vi "Constructor.vi"(8 "error in (no error)":errorcluster, 10 "FilePath":path, 11 "Name":string) -> (0 "error out":errorcluster, 3 "DocumentType out":refnum<class "Document.lvclass">)   [LabVIEW 2021, in "ProligentXMLGenerator.lvlib" / "Document.lvclass"]
uses:
  Document.lvclass
  Data.ctl
  CustomData/CustomData.lvclass
  Base/Guid/Guid.lvclass
  Base/NonEmptyString_255/NonEmptyString_255.lvclass
  Base/NonNullableString_600/NonNullableString_600.lvclass
  Document.lvclass/Document.ctl
  SetFilePath.vi
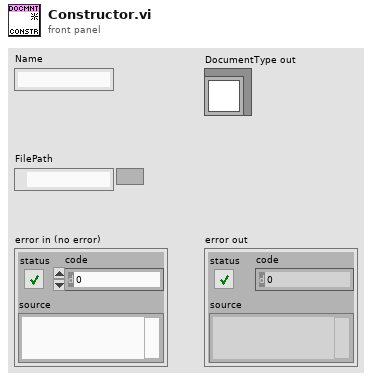
[diagram p1: front panel]
types:
  T1 = typedef "ProligentXMLGenerator.lvlib/Document.lvclass/Data.ctl" = cluster{"Name":string, "CustomData":refnum<class "CustomData.lvclass">, "Identifier":refnum<class "Guid.lvclass">, "NameType":refnum<class "NonEmptyString_255.lvclass">, "FileName":refnum<class "NonEmptyString_255.lvclass">, "Description":refnum<class "NonNullableString_600.lvclass">, "FilePath":path, "DestinationFolder":path}
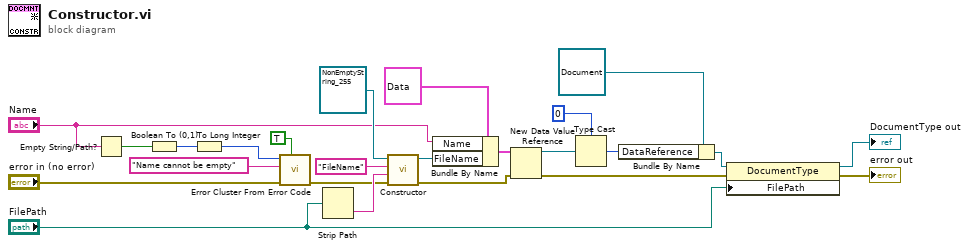
[diagram p0: block diagram]
diagram:
  n1 = Empty String/Path?(string/path="Name") -> (empty?=w24:bool)
  n2 = Boolean To (0,1)(Boolean=w24) -> (0, 1=w23:i16)
  n3 = To Long Integer(number=w23) -> (32bit integer=w17:i32)
  n4 = call <vilib>:"Error Cluster From Error Code.vi"("show call chain? (False)"=TRUE, "error in (no error)"="error in (no error)", "error message (\"\")"="Name cannot be empty" ("error message (\"\")"), "error code (0)"=w17) -> ("error out"=w13:errorcluster)  [unwired: 5 in]
  n5 = Strip Path(path="FilePath") -> (name=w18:string)  [unwired: 1 out]
  n6 = call-dynamic "Constructor.vi"("error in"=w13, "Value"=w18, "Name"="FileName", "String in"=refnum<class "NonEmptyString_255.lvclass"> refnum ("ProligentResultProcessor:NonEmptyString_255")) -> ("error out"=w3:errorcluster, "String out"=w21:refnum<class "NonEmptyString_255.lvclass">)  [unwired: 6 in]
  n7 = Bundle By Name(cluster=T1 {"Name"="", "CustomData"=refnum, "Identifier"=refnum, "NameType"=refnum, "FileName"=refnum, "Description"=refnum, "FilePath"=path "", "DestinationFolder"=path ""} ("Data"), "Name"="Name", "FileName"=w21) -> (w12:T1)
  n8 = New Data Value Reference(data value=w12, error in=w3) -> (data value reference=w11:refnum<data-value>, error out=w2:errorcluster)
  n9 = Type Cast(type=u64 0, x=w11) -> (*(type *) &x=w8:u64)
  n10 = Bundle By Name(cluster=refnum<class "Document.lvclass"> refnum ("ProligentResultProcessor:DocumentType"), "DataReference"=w8) -> (w7:refnum<class "Document.lvclass">)
  n11 = property class="DocumentType"(reference=w7, error in=w2, "FilePath"="FilePath") -> (reference out=→"DocumentType out":refnum<class "Document.lvclass">, error out=→"error out":errorcluster)
